vi "Write Sequence Config.lvclass.vi"(8 "error in (no error)":errorcluster, 10 "Sequence Config.lvclass":refnum<class "Sequence Config.lvclass">, 11 "SequenceNode in":refnum<class "SequenceNode.lvclass">) -> (0 "error out":errorcluster, 3 "SequenceNode out":refnum<class "SequenceNode.lvclass">)   [LabVIEW 2015, in "SequenceNode.lvclass"]
uses:
  SequenceNode.lvclass
  Prototype/classes/Sequence/Config/Sequence Config.lvclass
  SequenceNode.lvclass/SequenceNode.ctl
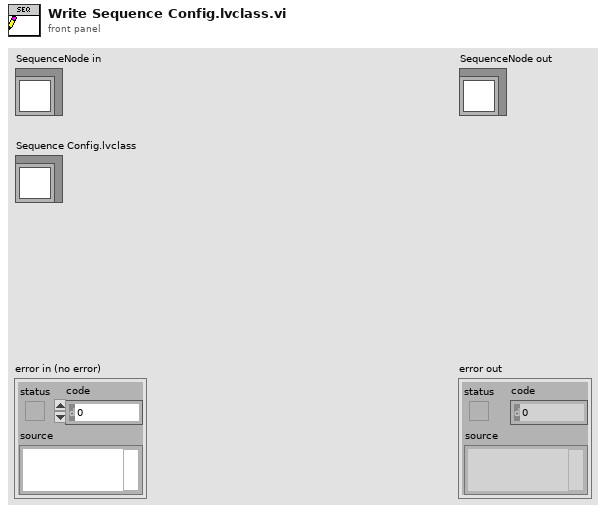
[diagram p1: front panel]
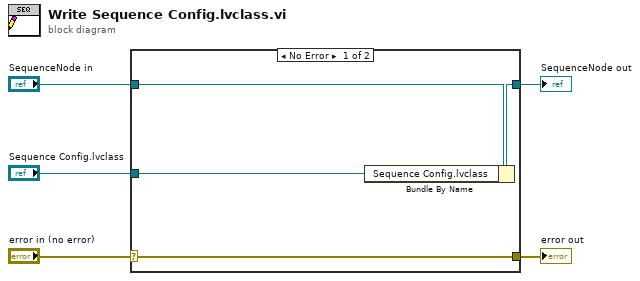
[diagram p0: block diagram]
diagram:
  n1 = case shown="No Error" "error in (no error)" {
    selector: "error in (no error)" -> [w9 w10]
    tunnel: [w9 w10] -> w4
    tunnel: [w7 w11] -> w2
    tunnel: "SequenceNode in" -> [w8 w11]
    tunnel: "Sequence Config.lvclass" -> [w6 _]
    frame No Error {
      n2 = Bundle By Name(cluster=w8, "Sequence Config.lvclass"=w6) -> (w7:refnum<class "SequenceNode.lvclass">)
    }
    frame Error {
    }
  }
  "error out" <- w4
  "SequenceNode out" <- w2
